vi "Create3DArray.vi"(11 "Position":dbl[](array[numeric])) -> (3 "3D Plot lvclass Array out":refnum<class "3D Plot Datatype.lvclass">[](array[class]))   [LabVIEW 2014, in "Serial Controller.lvclass"]
uses:
  Serial Controller.lvclass
  <vilib>/Math Plots/3D Math Plots/3D Plot/3D Plot Datatype/3D Plot Datatype.lvclass
  <vilib>/Math Plots/3D Math Plots/3D Scatter/3D Scatter Datatype/Public/Plot Helper (Vector).vi
  <vilib>/Math Plots/3D Math Plots/3D Scatter/3D Scatter Datatype/3D Scatter Datatype.lvclass
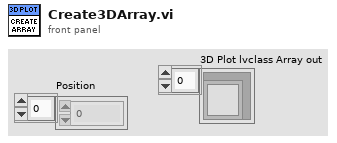
[diagram p1: front panel]
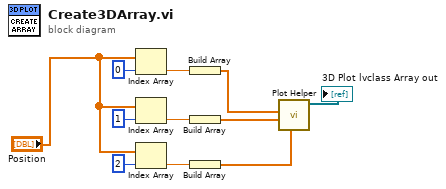
[diagram p0: block diagram]
diagram:
  n1 = Index Array(array="Position", index=0) -> (element=w9:dbl)
  n2 = Index Array(array="Position", index=1) -> (element=w10:dbl)
  n3 = Index Array(array="Position", index=2) -> (element=w11:dbl)
  n4 = Build Array(w9) -> (w5:dbl[])
  n5 = Build Array(w10) -> (w6:dbl[])
  n6 = Build Array(w11) -> (w7:dbl[])
  n7 = call-poly <vilib>:"Plot Helper.vi"("z vector"=w7, "y vector"=w6, "x vector"=w5) -> ("3D Plot lvclass Array out"=→"3D Plot lvclass Array out":refnum<class "3D Plot Datatype.lvclass">[])  [unwired: 3 in, 5 out]
